vi "SwerveModuleState_Optimize.vi"(9 "CurrentAngle":T1={"VALUE"=0.0, "COS"=1.0, "SIN"=0.0} {"SIN" format="%13.4f"; "COS" format="%13.4f"; "VALUE" format="%13.4f"}, 11 "Desired State":T2={"Speed"=0.0, "Angle"={"VALUE"=0.0, "COS"=1.0, "SIN"=0.0}} {"Angle"."SIN" format="%13.4f"; "Angle"."COS" format="%13.4f"; "Angle"."VALUE" format="%13.4f"}) -> (3 "out SWERVE_DRIVE_MODULE_STATE":T2={"Speed"=0.0, "Angle"={"VALUE"=0.0, "COS"=1.0, "SIN"=0.0}} {"Angle"."SIN" format="%13.4f"; "Angle"."COS" format="%13.4f"; "Angle"."VALUE" format="%13.4f"})   [LabVIEW 2019, in "Trajectory_Library.lvlib"]
doc: "Minimize the change in heading the desired swerve module state would require by potentially reversing the direction the wheel spins. If this is used with the PIDController class's continuous input functionality, the furthest a wheel will ever rotate is 90 degrees.\n\nParmeters:\n - desired Module State\n - current module angle (rotation)\n\nReturns:\n - optimized Module State"
uses:
  Trajectory_Library.lvlib
  TypeDef/ROTATION2D.ctl
  TypeDef/SWERVE_DRIVE_MODULE_STATE.ctl
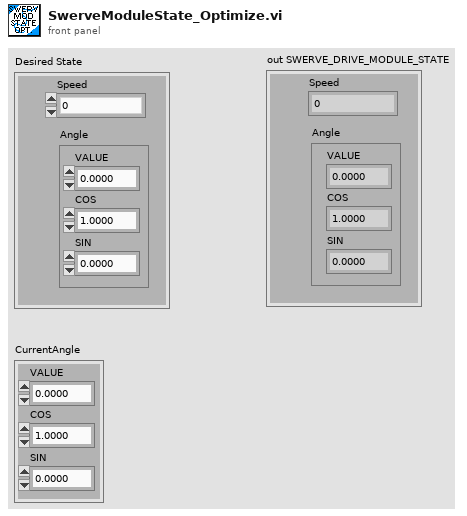
[diagram p1: front panel]
types:
  T1 = typedef "Trajectory_Library.lvlib/ROTATION2D.ctl" = cluster{"VALUE":dbl, "COS":dbl, "SIN":dbl}
  T2 = typedef "Trajectory_Library.lvlib/SWERVE_DRIVE_MODULE_STATE.ctl" = cluster{"Speed":dbl, "Angle":T1}
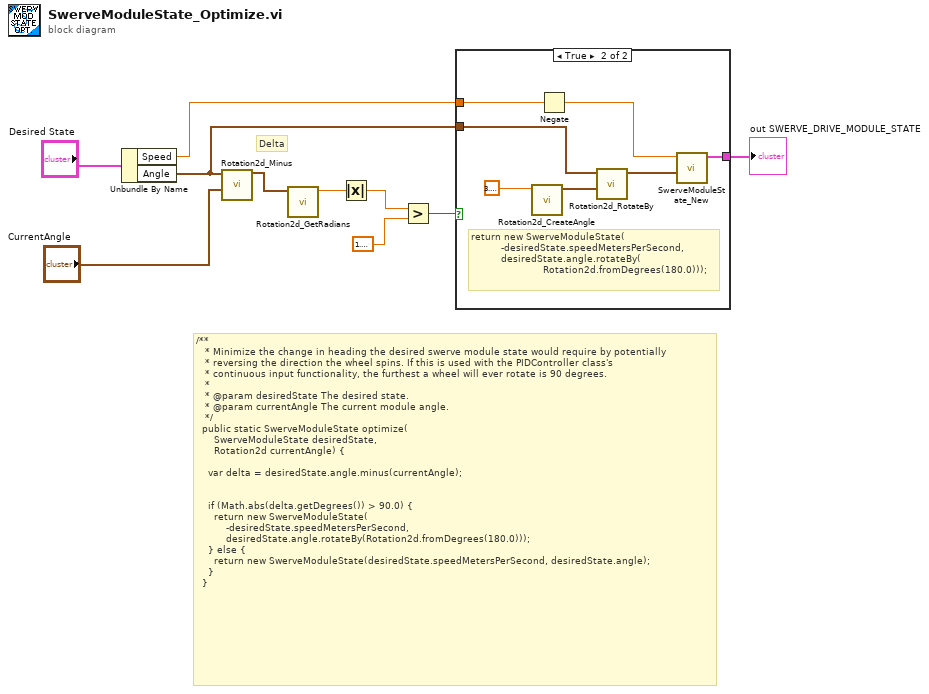
[diagram p0: block diagram]
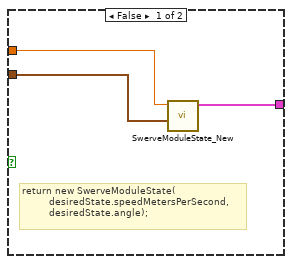
[diagram p2: hidden frame]
diagram:
  # "Delta"
  # "/**\n   * Minimize the change in heading the desired swerve module state would require by potentially\n   * reversing the direction the wheel spins. If this is used with the PIDController class's\n   * continuous input functionality, the furthest a wheel will ever rotate is 90 degrees.\n   *\n   * @param desiredState The desired state.\n   * @param currentAngle The current module angle.\n   */\n  public static SwerveModuleState optimize(\n      SwerveModuleState desiredState, \n      Rotation2d currentAngle) {\n\n    var delta = desiredState.angle.minus(currentAngle);\n\n\n    if (Math.abs(delta.getDegrees()) > 90.0) {\n      return new SwerveModuleState(\n          -desiredState.speedMetersPerSecond,\n          desiredState.angle.rotateBy(Rotation2d.fromDegrees(180.0)));\n    } else {\n      return new SwerveModuleState(desiredState.speedMetersPerSecond, desiredState.angle);\n    }\n  }"
  n1 = Unbundle By Name("Desired State") -> ("Speed"=w4:dbl, "Angle"=w3:T1)
  n2 = call "Rotation2d_Minus.vi"("other ROTATION"="CurrentAngle", "in ROTATION"=w3) -> ("out ROTATION"=w8:T1)  [unwired: 9 in]
  n3 = call "Rotation2d_GetRadians.vi"("in ROTATION"=w8) -> ("AngleRadians"=w2:dbl)  [unwired: 10 in]
  n4 = Absolute Value(x=w2) -> (abs(x)=w1:dbl)
  n5 = Greater?(x=w1, y=1.5707963267948966) -> (0:w6:bool)
  n6 = case shown="True" w6 {
    tunnel: [w13 w20] -> w5
    tunnel: w4 -> [w12 w19]
    tunnel: w3 -> [w11 w17]
    frame False {
      # "return new SwerveModuleState(\n         desiredState.speedMetersPerSecond, \n         desiredState.angle);"
      n7 = call "SwerveModuleState_New.vi"("ROTATION"=w11, "Speed"=w12) -> ("SWERVE_DRIVE_MODULE_STATE"=w13:T2)  [unwired: 9 in]
    }
    frame True {
      # "return new SwerveModuleState(\n          -desiredState.speedMetersPerSecond,\n          desiredState.angle.rotateBy(\n                        Rotation2d.fromDegrees(180.0)));"
      n8 = call "Rotation2d_CreateAngle.vi"("Angle"=3.141592653589793) -> ("ROTATION"=w14:T1)  [unwired: 10 in]
      n9 = Negate(x=w19) -> (-x=w18:dbl)
      n10 = call "Rotation2d_RotateBy.vi"("other Rotation"=w14, "in ROTATION"=w17) -> ("out ROTATION"=w16:T1)  [unwired: 9 in]
      n11 = call "SwerveModuleState_New.vi"("ROTATION"=w16, "Speed"=w18) -> ("SWERVE_DRIVE_MODULE_STATE"=w20:T2)  [unwired: 9 in]
    }
  }
  "out SWERVE_DRIVE_MODULE_STATE" <- w5
